vi "AAL Kaiser Parameters.vi"(8 "A stop [dB]":dbl=72.0 format="%.2f", 10 "delta f":dbl=0.1 format="%.2f", 11 "fs":dbl=1.0 format="%.2f") -> (0 "beta":dbl format="%.2f", 3 "taps":i32)   [LabVIEW 2010, in "NI_AALPro.lvlib"]
uses:
  NI_AALPro.lvlib
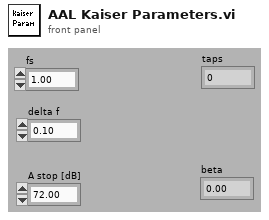
[diagram p1: front panel]
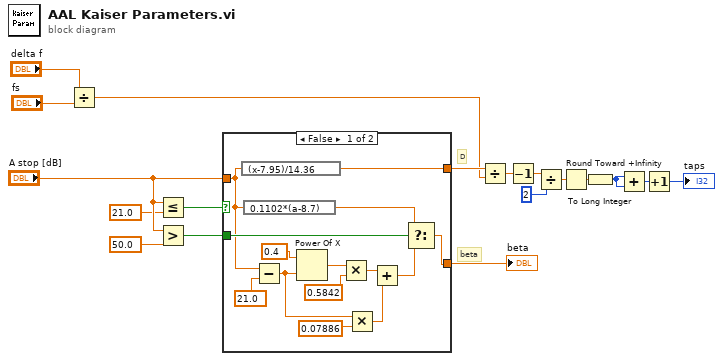
[diagram p0: block diagram]
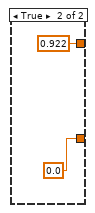
[diagram p2: hidden frame]
diagram:
  # "D"
  # "beta"
  n1 = Divide(x="delta f", y="fs") -> (x/y=w6:dbl)
  n2 = Less Or Equal?(x="A stop [dB]", y=21.0) -> (x <= y?=w12:bool)
  n3 = Greater?(x="A stop [dB]", y=50.0) -> (0:w13:bool)
  n4 = case shown="False" w12 {
    tunnel: [w31 0.0] -> w17
    tunnel: [w32 0.922] -> w7
    tunnel: w13 -> [w30 _]
    tunnel: "A stop [dB]" -> [w28 _]
    frame False {
      n5 = expression code="(x-7.95)/14.36"(w28) -> (w32:dbl)
      n6 = expression code="0.1102*(a-8.7)"(w28) -> (w29:dbl)
      n7 = Subtract(x=w28, y=21.0) -> (x-y=w22:dbl)
      n8 = Power Of X(1:w22, 2:0.4 ("y")) -> (0:w25:dbl)
      n9 = Multiply(x=w25, y=0.5842) -> (x*y=w21:dbl)
      n10 = Multiply(x=w22, y=0.07886) -> (x*y=w20:dbl)
      n11 = Add(x=w21, y=w20) -> (x+y=w19:dbl)
      n12 = Select(t=w29, s=w30, f=w19) -> (s? t:f=w31:dbl)
    }
    frame True {
    }
  }
  "beta" <- w17
  n13 = Divide(x=w7, y=w6) -> (x/y=w5:dbl)
  n14 = Decrement(x=w5) -> (x-1=w1:dbl)
  n15 = Divide(x=w1, y=2) -> (x/y=w15:dbl)
  n16 = Round Toward +Infinity(x=w15) -> (ceil(x): smallest int >= x=w16:dbl)
  n17 = To Long Integer(number=w16) -> (32bit integer=w3:i32)
  n18 = Add(x=w3, y=w3) -> (x+y=w4:i32)
  n19 = Increment(x=w4) -> (x+1=→"taps":i32)
